vi "Filter Log Packet.vi"(10 "Log Packet":T1, 11 "Compound Filter in":refnum<class "Compound Filter.lvclass">) -> (2 "Log?":bool, 3 "Compound Filter out":refnum<class "Compound Filter.lvclass">)   [LabVIEW 2017, in "Compound Filter.lvclass"]
uses:
  Compound Filter.lvclass
  Composed Log/Types/Log Packet.ctl
  Composed Log/Types/Log Level.ctl
  Compound Filter.lvclass/Compound Filter.ctl
  Composed Log/ILogFilter/ILogFilter.lvclass
  Composed Log/Composed Log.lvlib
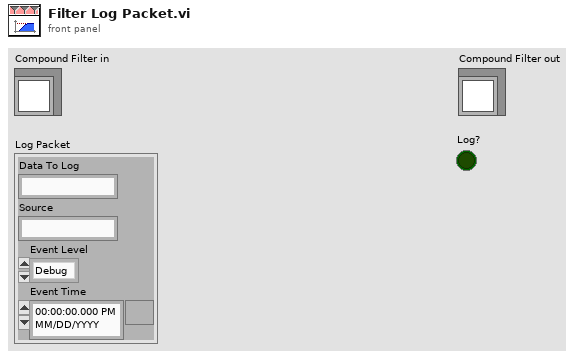
[diagram p1: front panel]
types:
  T1 = typedef "Composed Log.lvlib/Log Packet.ctl" = cluster{"Data To Log":string, "Source":string, "Event Level":T2, "Event Time":timestamp}
  T2 = typedef "Composed Log.lvlib/Log Level.ctl" = enum16{"Debug", "Info", "Warning", "Error", "Critical"}
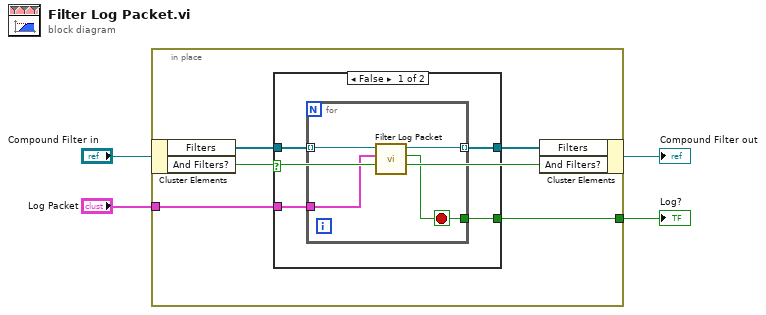
[diagram p0: block diagram]
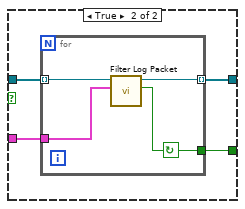
[diagram p2: hidden frame]
diagram:
  n1 = in-place {
    in-place-border: [w9] -> w4
    in-place-border: "Log Packet" -> [w8]
    n2 = in-place-cluster #1("Compound Filter in") -> ("Filters"=w7:refnum<class "ILogFilter.lvclass">[], "And Filters?"=w5:bool)
    n3 = case shown="False" w5 {
      tunnel: [w10 w21] -> w9
      tunnel: w8 -> [w12 w20]
      tunnel: w7 -> [w13 w19]
      tunnel: [w11 w18] -> w6
      frame False {
        n4 = for {
          tunnel: [w14] -> w10
          tunnel: w12 -> [w16]
          tunnel: w13 -> [w17] mode=indexing
          tunnel: [w15] -> w11 mode=indexing
          stop <- w14 stop-if-true
          n5 = call-dynamic "Filter Log Packet.vi"("Log Packet"=w16, "ILogFilter in"=w17) -> ("Log?"=w14:bool, "ILogFilter out"=w15:refnum<class "ILogFilter.lvclass">)  [unwired: 8 in]
        }
      }
      frame True {
        n6 = for {
          tunnel: [w23] -> w21
          tunnel: w20 -> [w24]
          tunnel: w19 -> [w25] mode=indexing
          tunnel: [w22] -> w18 mode=indexing
          stop <- w23 continue-if-true
          n7 = call-dynamic "Filter Log Packet.vi"("Log Packet"=w24, "ILogFilter in"=w25) -> ("Log?"=w23:bool, "ILogFilter out"=w22:refnum<class "ILogFilter.lvclass">)  [unwired: 8 in]
        }
      }
    }
    n8 = in-place-cluster #1("Filters"=w6, "And Filters?"=w5) -> (→"Compound Filter out":refnum<class "Compound Filter.lvclass">)
  }
  "Log?" <- w4
